vi "内部参数读写.vi"(11 "参数":enum16{"氨氮", "总磷", "总氮", "CODMn", "CODcr"}(ring)) -> ()   [LabVIEW 2016]
panel:
  in  "关闭":bool
  in  "写入参数":bool
  in  "读取参数":bool
  out "排液时间":u16
  out "搅拌时间":u16
  out "进样超时时间":u16
  out "润洗超时时间":u16
  out "润洗排液时间2":u16
  out "润洗排液时间1":u16
  out "润洗进样时间":u16
  # "内部参数"
  # "(0.1S,默认300)"
  # "(0.1S,默认500)"
  # "(0.1S,默认1400)"
  # "(0.1S,默认5000)"
  # "(0.1S,默认5000)"
  # "(0.1S,默认600)"
  # "(0.1S,默认1400)"
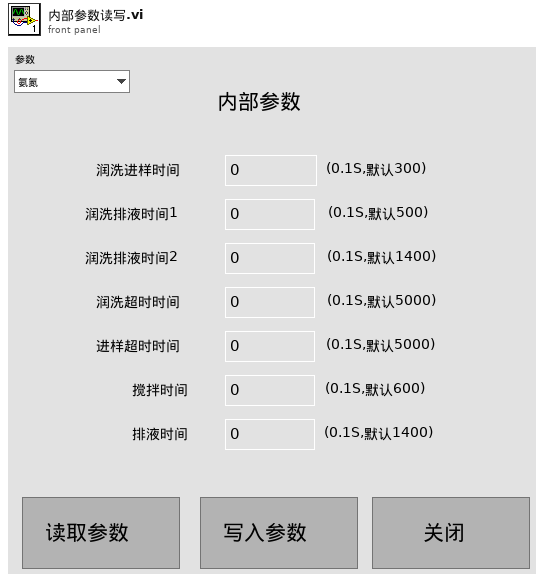
[diagram p1: front panel]
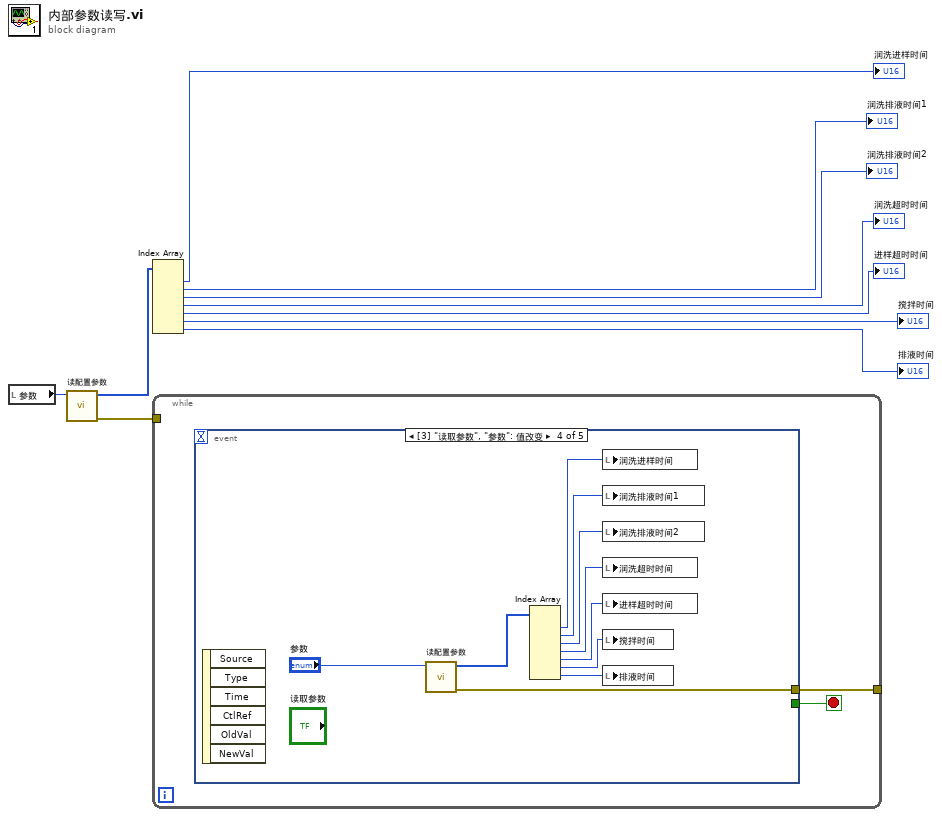
[diagram p0: block diagram]
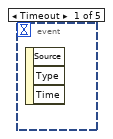
[diagram p2: hidden frame]
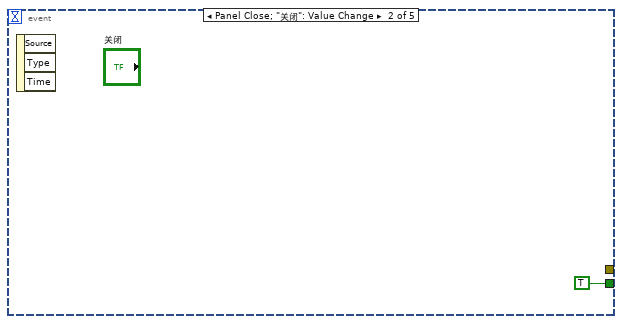
[diagram p3: hidden frame]
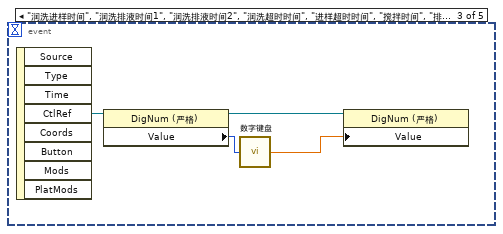
[diagram p4: hidden frame]
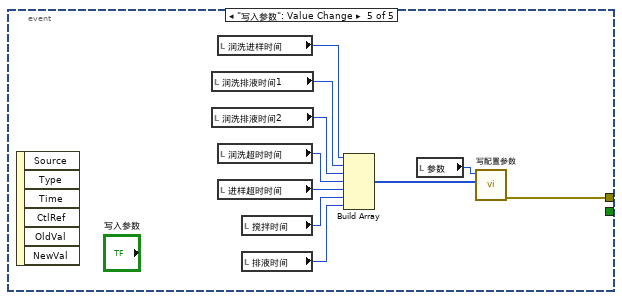
[diagram p5: hidden frame]
diagram:
  n1 = local read "参数"() -> (w2:enum16{"氨氮", "总磷", "总氮", "CODMn", "CODcr"})
  n2 = call "读配置参数.vi"("参数"=w2) -> ("error out"=w1:errorcluster, "values"=w10:u16[])  [unwired: 9 in]
  n3 = Index Array(array=w10) -> (element #1=→"润洗进样时间":u16, element #2=→"润洗排液时间1":u16, element #3=→"润洗排液时间2":u16, element #4=→"润洗超时时间":u16, element #5=→"进样超时时间":u16, element #6=→"搅拌时间":u16, element #7=→"排液时间":u16)  [unwired: 7 in]
  n4 = while {
    tunnel: [w11] -> _
    tunnel: w1 -> [_]
    stop <- w12 stop-if-true
    n5 = event shown="[3] \"读取参数\", \"参数\": 值改变" {
      selector: _ -> [_ _ _ _ _]
      dyn-events: _ -> [_ _ _ _ _]
      timeout: _ -> [_ _ _ _ _]
      tunnel: [_ TRUE _ _ _] -> w12
      tunnel: [_ _ _ w18 w28] -> w11
      event Timeout {
        n6 = event-data() -> ()  [unwired: 1 in, 3 out]
      }
      event Panel Close; "关闭": Value Change {
        n7 = event-data() -> ()  [unwired: 1 in, 3 out]
      }
      event "润洗进样时间", "润洗排液时间1", "润洗排液时间2", "润洗超时时间", "进样超时时间", "搅拌时间", "排液时间": Mouse Down {
        n8 = event-data() -> ("CtlRef"=w17:refnum<vi>)  [unwired: 1 in, 7 out]
        n9 = property class="DigNum (严格)"(reference=w17) -> (reference out=w15:refnum<vi>, "Value"=w16:u16)  [unwired: 1 in, 1 out]
        n10 = call "数字键盘.vi"("OldNumber"=w16) -> ("NewNumber"=w14:sgl)
        n11 = property class="DigNum (严格)"(reference=w15, "Value"=w14) -> ()  [unwired: 1 in, 2 out]
      }
      event "读取参数", "参数": Value Change {
        n12 = event-data() -> ()  [unwired: 1 in, 6 out]
        n13 = call "读配置参数.vi"("参数"="参数") -> ("error out"=w18:errorcluster, "values"=w26:u16[])  [unwired: 9 in]
        n14 = Index Array(array=w26) -> (element #1=w25:u16, element #2=w24:u16, element #3=w23:u16, element #4=w22:u16, element #5=w21:u16, element #6=w20:u16, element #7=w19:u16)  [unwired: 7 in]
        n15 = local write "润洗进样时间"(w25) -> ()
        n16 = local write "润洗排液时间1"(w24) -> ()
        n17 = local write "润洗排液时间2"(w23) -> ()
        n18 = local write "润洗超时时间"(w22) -> ()
        n19 = local write "进样超时时间"(w21) -> ()
        n20 = local write "搅拌时间"(w20) -> ()
        n21 = local write "排液时间"(w19) -> ()
      }
      event "写入参数": Value Change {
        n22 = event-data() -> ()  [unwired: 1 in, 6 out]
        n23 = local read "润洗排液时间1"() -> (w35:u16)
        n24 = local read "润洗排液时间2"() -> (w34:u16)
        n25 = local read "润洗进样时间"() -> (w36:u16)
        n26 = local read "润洗超时时间"() -> (w33:u16)
        n27 = local read "进样超时时间"() -> (w32:u16)
        n28 = local read "搅拌时间"() -> (w30:u16)
        n29 = local read "排液时间"() -> (w31:u16)
        n30 = Build Array(w36, w35, w34, w33, w32, w30, w31) -> (w29:u16[])
        n31 = local read "参数"() -> (w37:enum16{"氨氮", "总磷", "总氮", "CODMn", "CODcr"})
        n32 = call "写配置参数.vi"("values"=w29, "参数"=w37) -> ("error out"=w28:errorcluster)  [unwired: 9 in]
      }
    }
  }
